vi "BezahlSimulation.vi"(8 "error in (no error)":errorcluster) -> (0 "error out":errorcluster, 2 "Betrag erreicht":bool)   [LabVIEW 2023]
doc: "Bezahlsimulation\nerstellt: DI FH Mst Werner Bischof\nDatum: 22.10.2025"
uses:
  CONTROLS/fgv status.ctl
panel:
  out "Preis":dbl
  out "Restgeldausgabe":dbl
  in  "Storno":bool
  out "Guthaben":dbl
  in  "100Euro":bool
  in  "50Euro":bool
  in  "20Euro":bool
  in  "10Euro":bool
  in  "5Euro":bool
  in  "2Euro":bool
  in  "Bezahlen":bool
  in  "1Euro":bool
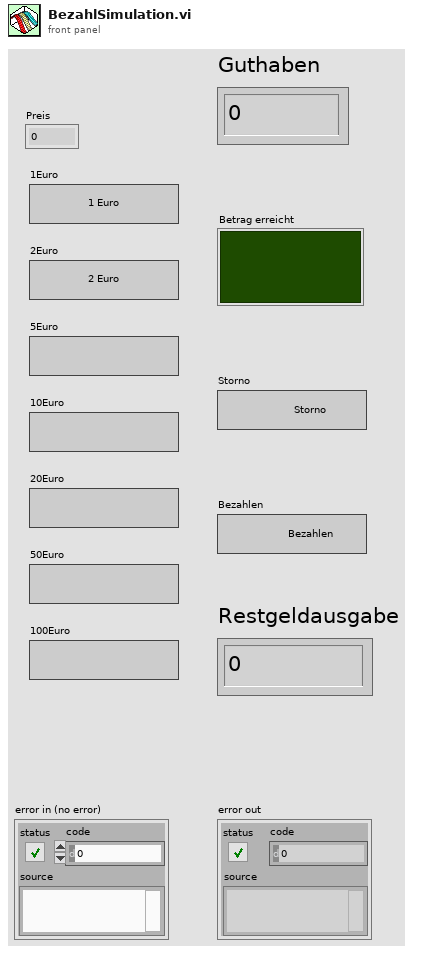
[diagram p1: front panel]
types:
  T1 = typedef "fgv status.ctl" = enum16{"Read", "Write"}
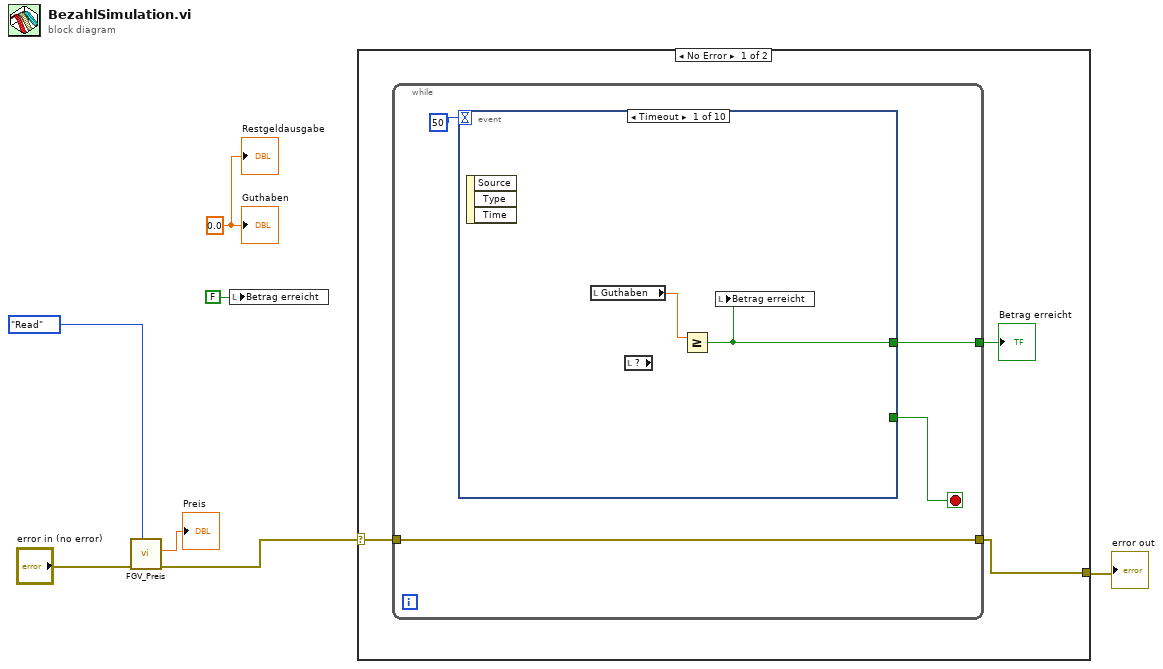
[diagram p0: block diagram]
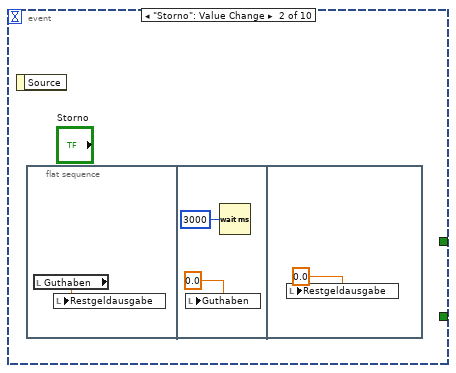
[diagram p2: hidden frame]
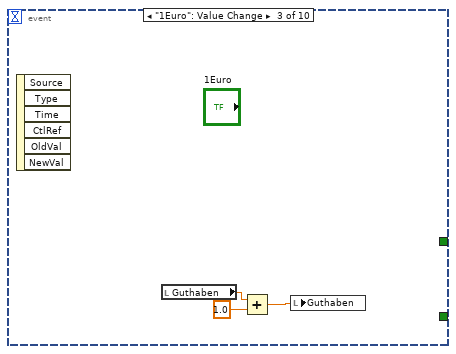
[diagram p3: hidden frame]
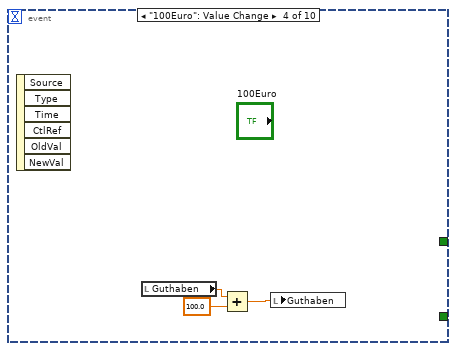
[diagram p4: hidden frame]
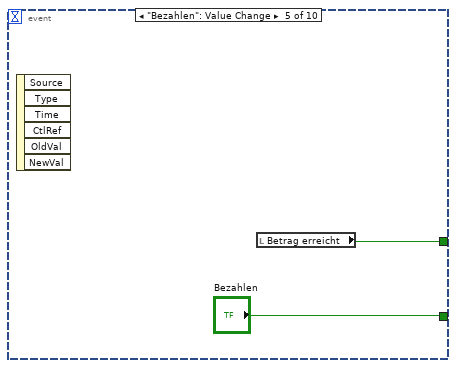
[diagram p5: hidden frame]
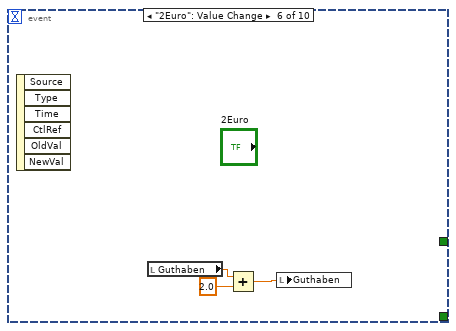
[diagram p6: hidden frame]
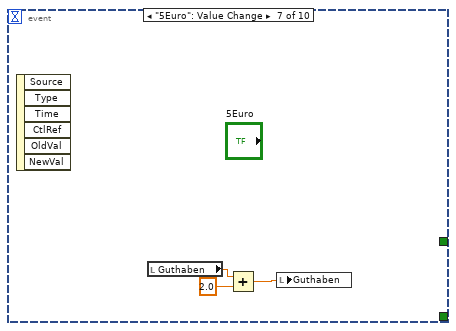
[diagram p7: hidden frame]
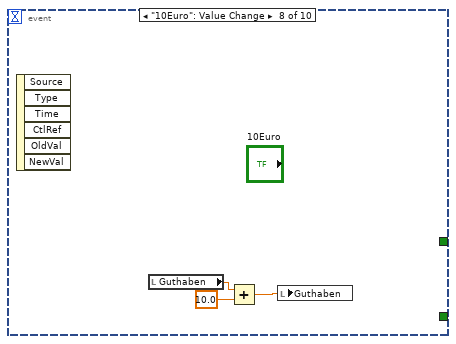
[diagram p8: hidden frame]
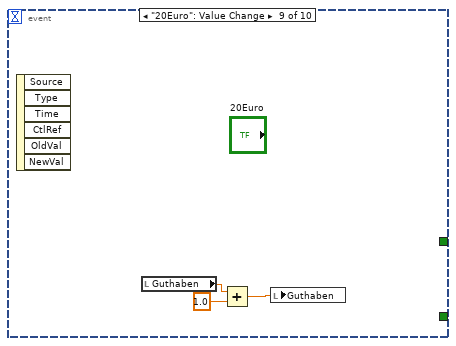
[diagram p9: hidden frame]
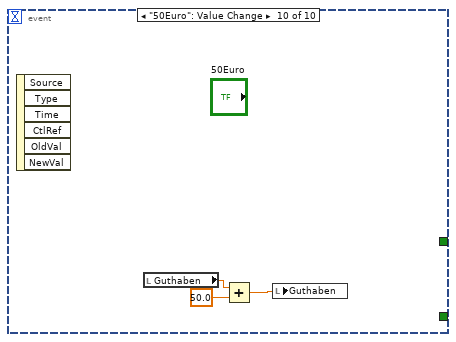
[diagram p10: hidden frame]
diagram:
  w6 = 0.0 ("Guthaben")
  n1 = call "FGV_Preis.vi"("FGV-Status"=fgv_status."Read", "error in (no error)"="error in (no error)") -> ("error out"=w3:errorcluster, "Preis Output"=→"Preis":dbl)  [unwired: 8 in]
  n2 = local write "Betrag erreicht"(FALSE ("Betrag erreicht")) -> ()
  n3 = case shown="No Error" w3 {
    selector: w3 -> [w9 _]
    tunnel: [w8 _] -> w2
    frame No Error {
      n4 = while {
        tunnel: [w12] -> w10
        tunnel: w9 -> [w11]
        tunnel: [w11] -> w8
        stop <- w14 stop-if-true
        n5 = event shown="[0] Timeout" {
          selector: _ -> [_ _ _ _ _ _ _ _ _ _]
          dyn-events: _ -> [_ _ _ _ _ _ _ _ _ _]
          timeout: 50 -> [_ _ _ _ _ _ _ _ _ _]
          tunnel: [_ _ _ _ "Bezahlen" _ _ _ _ _] -> w14
          tunnel: [w15 _ _ _ w27 _ _ _ _ _] -> w12
          event Timeout {
            n6 = event-data() -> ()  [unwired: 1 in, 3 out]
            n7 = local read "Guthaben"() -> (w16:dbl)
            n8 = local read item#-1() -> ()  [unwired: 1 out]
            n9 = Greater Or Equal?(x=w16) -> (x >= y?=w15:bool)  [unwired: 1 in]
            n10 = local write "Betrag erreicht"(w15) -> ()
          }
          event "Storno": Value Change {
            n11 = event-data() -> ()  [unwired: 1 in, 1 out]
            n12 = flat-sequence {
              frame #0 {
                n13 = local read "Guthaben"() -> (w17:dbl)
                n14 = local write "Restgeldausgabe"(w17) -> ()
              }
              frame #1 {
                n15 = local write "Guthaben"(0.0 ("Guthaben")) -> ()
                n16 = Wait (ms)(milliseconds to wait=u32 3000) -> ()  [unwired: 1 out]
              }
              frame #2 {
                n17 = local write "Restgeldausgabe"(0.0 ("Guthaben")) -> ()
              }
            }
          }
          event "1Euro": Value Change {
            n18 = event-data() -> ()  [unwired: 1 in, 6 out]
            n19 = local read "Guthaben"() -> (w23:dbl)
            n20 = Add(x=w23, y=1.0) -> (x+y=w22:dbl)
            n21 = local write "Guthaben"(w22) -> ()
          }
          event "100Euro": Value Change {
            n22 = event-data() -> ()  [unwired: 1 in, 6 out]
            n23 = local read "Guthaben"() -> (w26:dbl)
            n24 = Add(x=w26, y=100.0) -> (x+y=w25:dbl)
            n25 = local write "Guthaben"(w25) -> ()
          }
          event "Bezahlen": Value Change {
            n26 = event-data() -> ()  [unwired: 1 in, 6 out]
            n27 = local read "Betrag erreicht"() -> (w27:bool)
          }
          event "2Euro": Value Change {
            n28 = event-data() -> ()  [unwired: 1 in, 6 out]
            n29 = local read "Guthaben"() -> (w31:dbl)
            n30 = Add(x=w31, y=2.0) -> (x+y=w30:dbl)
            n31 = local write "Guthaben"(w30) -> ()
          }
          event "5Euro": Value Change {
            n32 = event-data() -> ()  [unwired: 1 in, 6 out]
            n33 = local read "Guthaben"() -> (w34:dbl)
            n34 = Add(x=w34, y=2.0) -> (x+y=w33:dbl)
            n35 = local write "Guthaben"(w33) -> ()
          }
          event "10Euro": Value Change {
            n36 = event-data() -> ()  [unwired: 1 in, 6 out]
            n37 = local read "Guthaben"() -> (w37:dbl)
            n38 = Add(x=w37, y=10.0) -> (x+y=w36:dbl)
            n39 = local write "Guthaben"(w36) -> ()
          }
          event "20Euro": Value Change {
            n40 = event-data() -> ()  [unwired: 1 in, 6 out]
            n41 = local read "Guthaben"() -> (w40:dbl)
            n42 = Add(x=w40, y=1.0) -> (x+y=w39:dbl)
            n43 = local write "Guthaben"(w39) -> ()
          }
          event "50Euro": Value Change {
            n44 = event-data() -> ()  [unwired: 1 in, 6 out]
            n45 = local read "Guthaben"() -> (w43:dbl)
            n46 = Add(x=w43, y=50.0) -> (x+y=w42:dbl)
            n47 = local write "Guthaben"(w42) -> ()
          }
        }
      }
      "Betrag erreicht" <- w10
    }
    frame Error {
    }
  }
  "error out" <- w2
  "Guthaben" <- w6
  "Restgeldausgabe" <- w6
